vi "WPI_SolenoidGetEnum.vi"(8 "error in (no error)":errorcluster, 11 "SolenoidDevRef":T2={"DevStatus"={"status"=FALSE, "code"=0, "source"=""}, "Pneumatics Control Module"=0, "Forward Solenoid Channel"=enum."Invalid", "Reverse Solenoid Channel"=enum."Invalid"}) -> (0 "error out":errorcluster, 2 "Value":T1, 3 "SolenoidDevRef":T2={"DevStatus"={"status"=FALSE, "code"=0, "source"=""}, "Pneumatics Control Module"=0, "Forward Solenoid Channel"=enum."Invalid", "Reverse Solenoid Channel"=enum."Invalid"})   [LabVIEW 2017]
doc: "Returns whether a Single solenoid is On or Off, or whether a Double solenoid is Forward, Reverse, or Off.\n\nThis software is licensed. Open the labview\\readme\\WPI Robotics Library Open Source License.txt file for more information."
uses:
  <vilib>/Rock Robotics/WPI/Solenoid/WPI_SolenoidDevRef.ctl
  <vilib>/Rock Robotics/WPI/Solenoid/WPI_SolenoidChannel.ctl
  <vilib>/Rock Robotics/WPI/Solenoid/WPI_SolenoidValue.ctl
  <vilib>/Rock Robotics/WPI/CAN/PCM/WPI_CAN_PCMGlobalOps.ctl
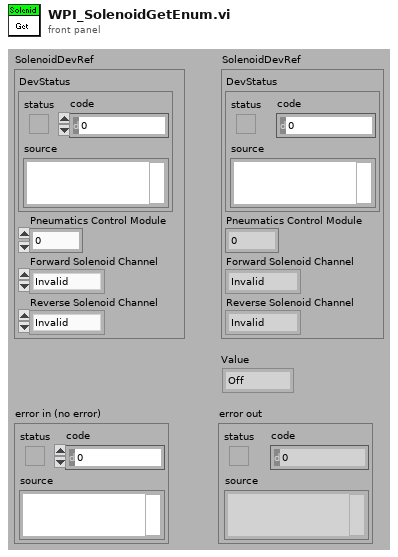
[diagram p1: front panel]
types:
  T1 = typedef "WPI_SolenoidValue.ctl" = enum16{"Off", "On", "Forward", "Reverse"}
  T2 = typedef "WPI_SolenoidDevRef.ctl" = cluster{"DevStatus":errorcluster, "Pneumatics Control Module":u8, "Forward Solenoid Channel":T3, "Reverse Solenoid Channel":T3}
  T3 = typedef "WPI_SolenoidChannel.ctl" = enum8{"Solenoid 0", "Solenoid 1", "Solenoid 2", "Solenoid 3", "Solenoid 4", "Solenoid 5", "Solenoid 6", "Solenoid 7", "Invalid"}
  T4 = typedef "WPI_CAN_PCMGlobalOps.ctl" = enum16{"Read For Send", "Write After Receive", "Set Solenoids", "Set Closed Loop", "Clear Sticky Faults", "Get All", "Write Error", "Write After Receive Blacklist", "Set Control Frame Rate"}
  T5 = cluster{"Solenoid Status":bool[], "Battery Voltage":dbl, "Solenoid Voltage":dbl, "Compressor Current":dbl, "CompressorEnabled":bool, "StickySolenoidFault":bool, "StickyCompressorFault":bool, "SolenoidFault":bool, "CompressorFault":bool, "HardwareFault":bool, "ClosedLoopStatus":bool, "PressureStatus":bool, "Module Enabled":bool, "ClosedLoopSuggestedOutput":bool, "CAN Error":errorcluster, "Sticky Solenoid Faults":bool[]}
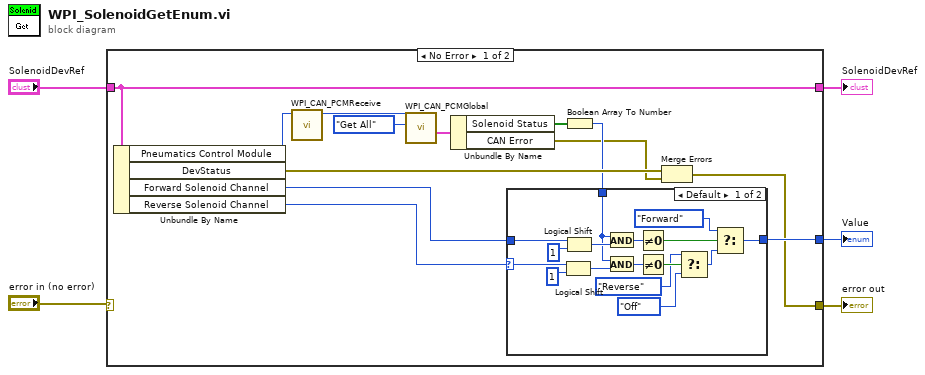
[diagram p0: block diagram]
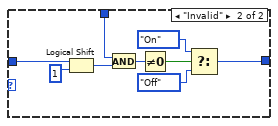
[diagram p2: hidden frame]
diagram:
  n1 = case shown="No Error" "error in (no error)" {
    selector: "error in (no error)" -> [_ w45]
    tunnel: "SolenoidDevRef" -> [w6 w44]
    tunnel: [w13 w45] -> w3
    tunnel: [w6 w44] -> w2
    tunnel: [w17 _] -> w1
    frame No Error {
      n2 = Unbundle By Name(w6) -> ("Pneumatics Control Module"=w8:u8, "DevStatus"=w15:errorcluster, "Forward Solenoid Channel"=w18:T3, "Reverse Solenoid Channel"=w16:T3)
      n3 = call <vilib>:"WPI_CAN_PCMReceive.vi"("Pneumatics Control Module (0)"=w8) -> ("Pneumatics Control Module Out"=w7:u8)  [unwired: 10 in]
      n4 = call <vilib>:"WPI_CAN_PCMGlobal.vi"("Operation"=WPI_CAN_PCMGlobalOps."Get All", "Pneumatics Control Module (0)"=w7) -> ("Get All"=w12:T5)  [unwired: 7 in, 2 out]
      n5 = Unbundle By Name(w12) -> ("Solenoid Status"=w11:bool[], "CAN Error"=w9:errorcluster)
      n6 = Boolean Array To Number(Boolean array=w11) -> (number=w10:u32)
      n7 = case shown="Default" w16 {
        selector: w16 -> [w28 _]
        tunnel: w18 -> [w33 w42]
        tunnel: w10 -> [w27 w41]
        tunnel: [w24 w37] -> w17
        frame Default {
          n8 = Logical Shift(y=w28, x=u8 1) -> (x << y=w26:u8)
          n9 = Logical Shift(y=w33, x=u8 1) -> (x << y=w32:u8)
          n10 = And(x=w27, y=w32) -> (x .and. y?=w31:u32)
          n11 = And(x=w27, y=w26) -> (x .and. y?=w25:u32)
          n12 = Not Equal To 0?(x=w31) -> (x != 0?=w30:bool)
          n13 = Not Equal To 0?(x=w25) -> (x != 0?=w23:bool)
          n14 = Select(t=WPI_SolenoidValue."Reverse" ("Value"), s=w23, f=WPI_SolenoidValue."Off" ("Value")) -> (s? t:f=w22:T1)
          n15 = Select(t=WPI_SolenoidValue."Forward" ("Value"), s=w30, f=w22) -> (s? t:f=w24:T1)
        }
        frame "Invalid" {
          n16 = Logical Shift(y=w42, x=u8 1) -> (x << y=w40:u8)
          n17 = And(x=w41, y=w40) -> (x .and. y?=w39:u32)
          n18 = Not Equal To 0?(x=w39) -> (x != 0?=w38:bool)
          n19 = Select(t=WPI_SolenoidValue."On" ("Value"), s=w38, f=WPI_SolenoidValue."Off" ("Value")) -> (s? t:f=w37:T1)
        }
      }
      n20 = Merge Errors(w15, w9) -> (w13:errorcluster)
    }
    frame Error {
    }
  }
  "SolenoidDevRef" <- w2
  "error out" <- w3
  "Value" <- w1
